vi "Modify_Image_Histogram-4.vi"(7 "1 - Origin\n2 - LoG":u8, 8 "error IN":errorcluster, 9 "[IN] Image Filtering Settings":T1, 11 "[IN] LoG Processed Image":T3) -> (0 "error OUT":errorcluster, 2 "[OUT] Histogram":T2 {"Incremental Value" format="%.2f"; "Starting Value" format="%.2f"}, 3 "[OUT] Histogram Modified Image":T3)   [LabVIEW 2013]
doc: "This subVI modifies image through various mathlookup operations (see the built-in function \"IMAQ MathLookup\")\nIn other words, it makes the gamma correction of picture (exchanging if intensity for each single pixel by multiplying of this pixel value on some function)"
uses:
  <vilib>/vision/Image Controls.llb/IMAQ Image.ctl
  <vilib>/vision/NI_Vision_Development_Module.lvlib
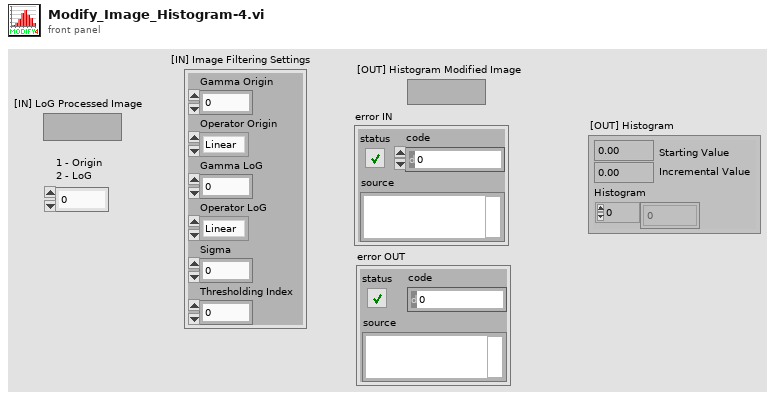
[diagram p1: front panel]
types:
  T1 = cluster{"Gamma Origin":sgl, "Operator Origin":enum32{"Linear", "Log", "Exp", "Square", "Square root", "Power X", "Power 1/X"}, "Gamma LoG":sgl, "Operator LoG":enum32{"Linear", "Log", "Exp", "Square", "Square root", "Power X", "Power 1/X"}, "Sigma":dbl, "Thresholding Index":i8}
  T2 = cluster{"Starting Value":sgl, "Incremental Value":sgl, "Histogram":u32[]}
  T3 = typedef "IMAQ Image.ctl" = refnum<image>
  T4 = enum32{"Linear", "Log", "Exp", "Square", "Square root", "Power X", "Power 1/X"}
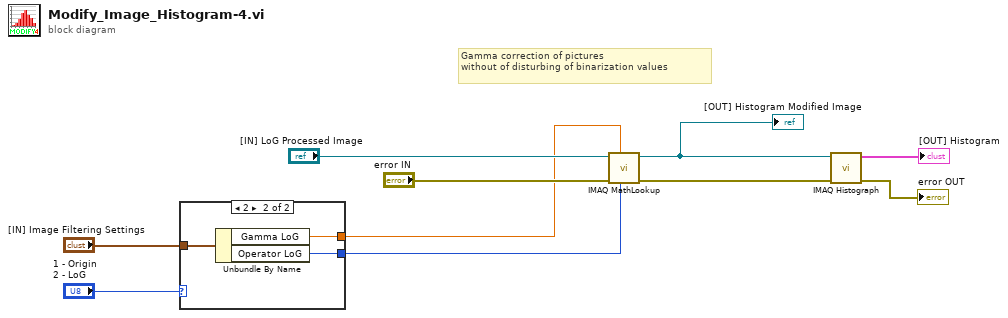
[diagram p0: block diagram]
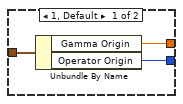
[diagram p2: hidden frame]
diagram:
  # "Gamma correction of pictures\nwithout of disturbing of binarization values"
  n1 = case shown="2" "1 - Origin\n2 - LoG" {
    tunnel: "[IN] Image Filtering Settings" -> [w13 w16]
    tunnel: [w12 w15] -> w2
    tunnel: [w11 w14] -> w1
    frame 1, Default {
      n2 = Unbundle By Name(w13) -> ("Gamma Origin"=w12:sgl, "Operator Origin"=w11:T4)
    }
    frame 2 {
      n3 = Unbundle By Name(w16) -> ("Gamma LoG"=w15:sgl, "Operator LoG"=w14:T4)
    }
  }
  n4 = call "IMAQ MathLookup"("Operator"=w1, "X Value"=w2, "error in (no error)"="error IN", "Image Src"="[IN] LoG Processed Image") -> ("error out"=w3:errorcluster, "Image Dst Out"=w7:T3)  [unwired: 6 in]
  "[OUT] Histogram Modified Image" <- w7
  n5 = call "IMAQ Histograph"("error in (no error)"=w3, "Image"=w7) -> ("error out"=→"error OUT":errorcluster, "Histogram Graph"=→"[OUT] Histogram":T2)  [unwired: 6 in, 2 out]
